vi "digital write.vi"() -> ()   [LabVIEW 2017]
uses:
  <vilib>/LabVIEW Interface for Arduino/Type Defs/Board Type.ctl
  <vilib>/LabVIEW Interface for Arduino/Type Defs/Connection Type.ctl
  <vilib>/LabVIEW Interface for Arduino/Type Defs/Pin Mode.ctl
  <vilib>/LabVIEW Interface for Arduino/LabVIEW Interface for Arduino.lvlib
panel:
  in  "Boolean":bool
  in  "Digital I/O Pin (0)":u8
  in  "milliseconds to wait":u32
  in  "Stop Button":bool
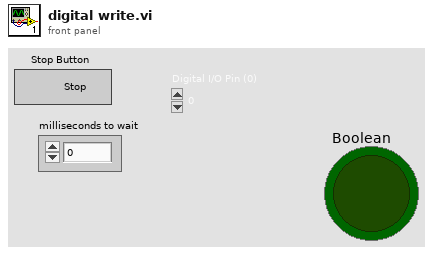
[diagram p1: front panel]
types:
  T1 = typedef "LabVIEW Interface for Arduino.lvlib/Connection Type.ctl" = enum8{"USB / Serial", "XBEE", "BlueSmirf (Bluetooth)"}
  T2 = typedef "LabVIEW Interface for Arduino.lvlib/Board Type.ctl" = enum16{"Uno", "Dimuelanove w/Atmega 328", "Mega 2560"}
  T3 = typedef "LabVIEW Interface for Arduino.lvlib/Arduino Resource.ctl" = cluster{"VISA resource":refnum<visa-resource-name>, "Board Type":T2, "Connection Type":enum8{"USB / Serial"}, "Bytes Per Packet (15)":u8}
  T4 = typedef "LabVIEW Interface for Arduino.lvlib/Pin Mode.ctl" = enum8{"Input", "Output"}
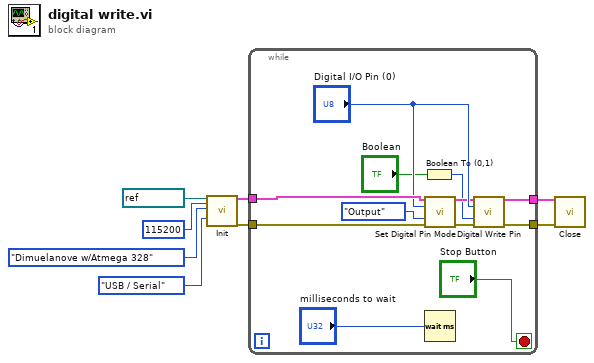
[diagram p0: block diagram]
diagram:
  n1 = call <vilib>:"Init.vi"("VISA resource"=refnum<visa-resource-name> "COM4", "Baud Rate (115200)"=u32 115200, "Board Type (Uno)"=Board_Type."Dimuelanove w/Atmega 328", "Connection Type (USB/Serial)"=Connection_Type."USB / Serial") -> ("Arduino Resource"=w4:T3, "error out"=w3:errorcluster)  [unwired: 14 in]
  n2 = while {
    tunnel: w4 -> [w19]
    tunnel: w3 -> [w18]
    tunnel: [w10] -> w2
    tunnel: [w9] -> w1
    stop <- "Stop Button" stop-if-true
    n3 = Boolean To (0,1)(Boolean="Boolean") -> (0, 1=w11:i16)
    n4 = call <vilib>:"Set Digital Pin Mode.vi"("Arduino Resource"=w19, "Digital I/O Pin"="Digital I/O Pin (0)", "Pin Mode (Input)"=Pin_Mode."Output", "error in"=w18) -> ("Arduino Resource"=w13:T3, "error out"=w15:errorcluster)  [unwired: 10 in]
    n5 = Wait (ms)(milliseconds to wait="milliseconds to wait") -> ()  [unwired: 1 out]
    n6 = call <vilib>:"Digital Write Pin.vi"("Arduino Resource"=w13, "Digital I/O Pin (0)"="Digital I/O Pin (0)", "Value (0)"=w11, "error in"=w15) -> ("Arduino Resource"=w10:T3, "error out"=w9:errorcluster)  [unwired: 10 in]
  }
  n7 = call <vilib>:"Close.vi"("Arduino Resource"=w2, "error in"=w1) -> ()  [unwired: 13 in, 1 out]
